vi "manualFreq.vi"(10 "Use DDS display equivalent?":bool, 11 "Manual Frequency (MHz)":dbl) -> (2 "DDS display value":u32, 3 "Frequency string out":string)   [LabVIEW 2012, in "DDS9954_v2013.lvlib"]
uses:
  DDS9954_v2013.lvlib
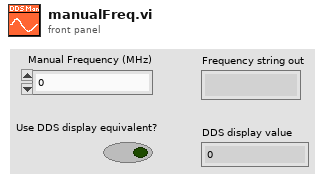
[diagram p1: front panel]
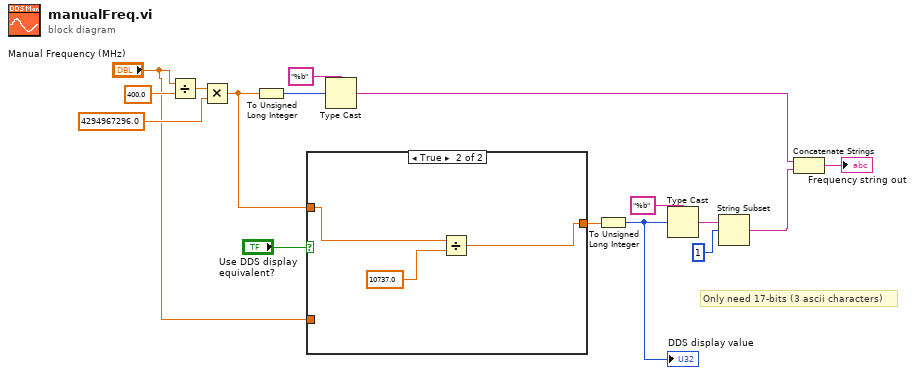
[diagram p0: block diagram]
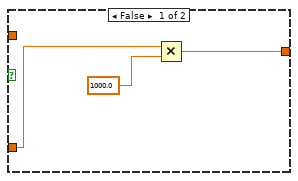
[diagram p2: hidden frame]
diagram:
  # "Only need 17-bits (3 ascii characters)"
  n1 = Divide(x="Manual Frequency (MHz)", y=400.0) -> (x/y=w13:dbl)
  n2 = Multiply(x=w13, y=4294967296.0) -> (x*y=w10:dbl)
  n3 = To Unsigned Long Integer(number=w10) -> (unsigned 32bit integer=w16:u32)
  n4 = case shown="True" "Use DDS display equivalent?" {
    tunnel: w10 -> [_ w22]
    tunnel: "Manual Frequency (MHz)" -> [w18 _]
    tunnel: [w17 w20] -> w6
    frame False {
      n5 = Multiply(x=w18, y=1000.0) -> (x*y=w17:dbl)
    }
    frame True {
      n6 = Divide(x=w22, y=10737.0) -> (x/y=w20:dbl)
    }
  }
  n7 = Type Cast(type="%b", x=w16) -> (*(type *) &x=w5:string)
  n8 = To Unsigned Long Integer(number=w6) -> (unsigned 32bit integer=w8:u32)
  "DDS display value" <- w8
  n9 = Type Cast(type="%b", x=w8) -> (*(type *) &x=w3:string)
  n10 = String Subset(string=w3, offset (0)=1) -> (substring=w1:string)  [unwired: 1 in]
  n11 = Concatenate Strings(w5, w1) -> (→"Frequency string out":string)
